vi "Pure Tones.vi"(0 "Amplitude (V)":dbl=1.0 max=19.0 step=1.0, 1 "Frequency (Hz)":dbl=4000.0 min=400.0 max=60000.0 step=10.0, 2 "Stimulation freq (stim/sec)":u32=20, 3 "Fs (#S/s)":dbl=200000.0) -> (4 "Signal duration (ms)":dbl, 5 "Stimulus Waveform":waveform(dbl)(graph), 6 "Stimulus duration (ms)":dbl, 7 "Delay (ms)":dbl=1.0, 8 "Signal duration (#S)":dbl)   [LabVIEW 2014]
uses:
  <vilib>/Analysis/1siggen.llb/Ramp Pattern by Samples.vi
  <vilib>/Analysis/NI_AALBase.lvlib
panel:
  out "Amplitude (1/10 V)":dbl
  out "Phase 1 (degrees)":dbl
  out "Plateu duration (#S)":dbl
  out "Ramp duration (#S)":dbl
  in  "start":dbl
  out "end":dbl
  out "Delay (#S)":dbl
  out "Frecuency (cycles/#S)":dbl
  in  "Plateu duration (ms)":dbl=10.0
  in  "Ramp duration (ms)":dbl=1.0
  # "Stimulus Configuration"
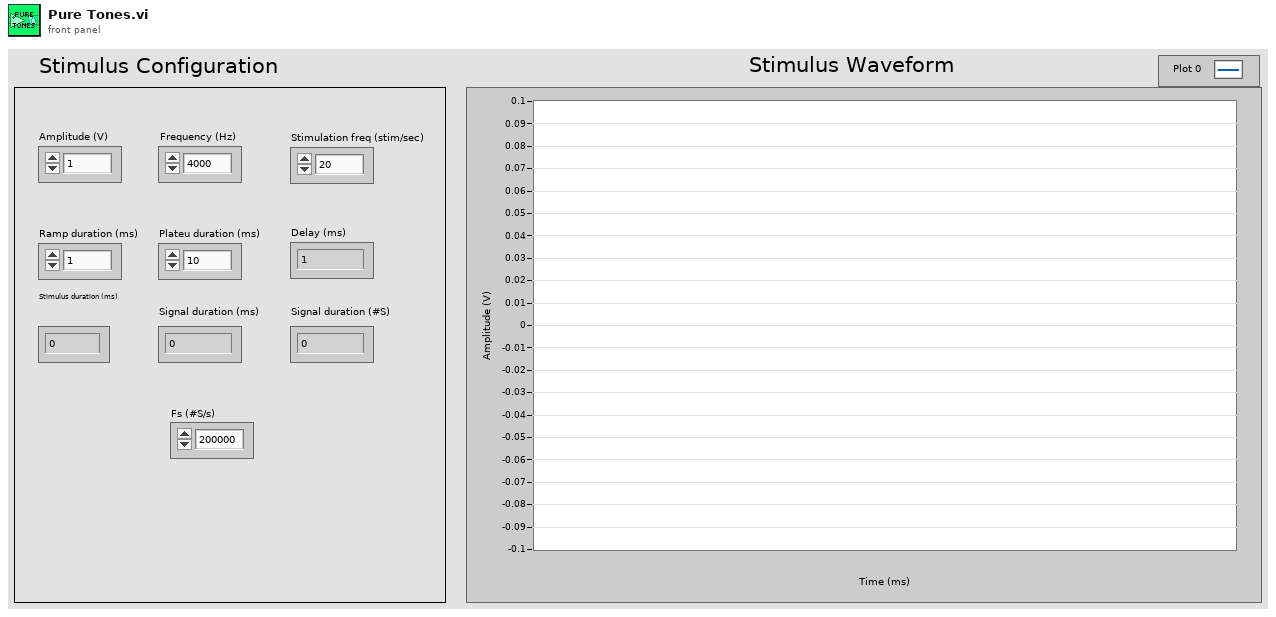
[diagram p1: front panel]
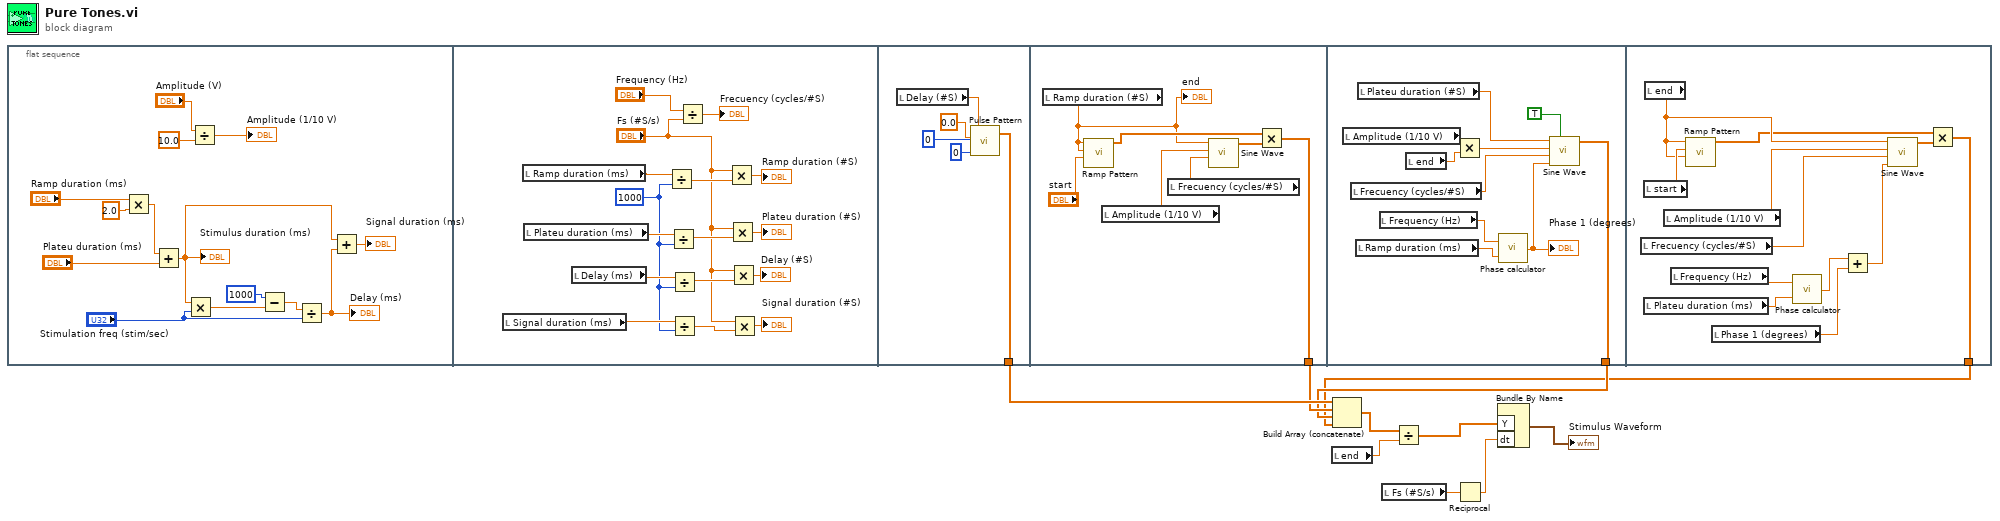
[diagram p0: block diagram]
diagram:
  n1 = flat-sequence {
    tunnel: [w41] -> w9
    tunnel: [w47] -> w8
    tunnel: [w53] -> w7
    tunnel: [w63] -> w6
    frame #0 {
      n2 = Multiply(x="Ramp duration (ms)", y=2.0) -> (x*y=w20:dbl)
      n3 = Add(x=w20, y="Plateu duration (ms)") -> (x+y=w12:dbl)
      "Stimulus duration (ms)" <- w12
      n4 = Multiply(x=w12, y="Stimulation freq (stim/sec)") -> (x*y=w16:dbl)
      n5 = Divide(x="Amplitude (V)", y=10.0) -> (x/y=→"Amplitude (1/10 V)":dbl)
      n6 = Subtract(x=1000, y=w16) -> (x-y=w15:dbl)
      n7 = Divide(x=w15, y="Stimulation freq (stim/sec)") -> (x/y=w11:dbl)
      "Delay (ms)" <- w11
      n8 = Add(x=w12, y=w11) -> (x+y=→"Signal duration (ms)":dbl)
    }
    frame #1 {
      w28 = 1000
      n9 = local read "Signal duration (ms)"() -> (w29:dbl)
      n10 = local read "Ramp duration (ms)"() -> (w38:dbl)
      n11 = local read "Plateu duration (ms)"() -> (w35:dbl)
      n12 = local read "Delay (ms)"() -> (w32:dbl)
      n13 = Divide(x=w38, y=w28) -> (x/y=w36:dbl)
      n14 = Divide(x=w35, y=w28) -> (x/y=w34:dbl)
      n15 = Divide(x=w32, y=w28) -> (x/y=w31:dbl)
      n16 = Divide(x=w29, y=w28) -> (x/y=w27:dbl)
      n17 = Divide(x="Frequency (Hz)", y="Fs (#S/s)") -> (x/y=→"Frecuency (cycles/#S)":dbl)
      n18 = Multiply(x="Fs (#S/s)", y=w36) -> (x*y=→"Ramp duration (#S)":dbl)
      n19 = Multiply(x="Fs (#S/s)", y=w34) -> (x*y=→"Plateu duration (#S)":dbl)
      n20 = Multiply(x="Fs (#S/s)", y=w31) -> (x*y=→"Delay (#S)":dbl)
      n21 = Multiply(x="Fs (#S/s)", y=w27) -> (x*y=→"Signal duration (#S)":dbl)
    }
    frame #2 {
      n22 = local read "Delay (#S)"() -> (w45:dbl)
      n23 = call <vilib>:"Pulse Pattern.vi"("width"=0, "delay"=0, "amplitude"=0.0, "samples"=w45) -> ("Pulse Pattern"=w41:dbl[])  [unwired: 1 out]
    }
    frame #3 {
      n24 = local read "Ramp duration (#S)"() -> (w46:dbl)
      "end" <- w46
      n25 = call-poly <vilib>:"Ramp Pattern.vi"("start"="start", "end"=w46, "samples"=w46) -> ("Ramp Pattern"=w48:dbl[])  [unwired: 7 in, 1 out]
      n26 = local read "Amplitude (1/10 V)"() -> (w50:dbl)
      n27 = local read "Frecuency (cycles/#S)"() -> (w51:dbl)
      n28 = call <vilib>:"Sine Wave.vi"("samples"=w46, "amplitude"=w50, "frequency"=w51) -> ("sine wave"=w49:dbl[])  [unwired: 2 in, 2 out]
      n29 = Multiply(x=w48, y=w49) -> (x*y=w47:dbl[])
    }
    frame #4 {
      n30 = local read "Amplitude (1/10 V)"() -> (w61:dbl)
      n31 = local read "Frecuency (cycles/#S)"() -> (w58:dbl)
      n32 = local read "Ramp duration (ms)"() -> (w56:dbl)
      n33 = local read "Plateu duration (#S)"() -> (w62:dbl)
      n34 = local read "Frequency (Hz)"() -> (w57:dbl)
      n35 = local read "end"() -> (w60:dbl)
      n36 = Multiply(x=w61, y=w60) -> (x*y=w59:dbl)
      n37 = call <userlib>:"Phase calculator.vi"("Frequency (Hz)"=w56, "Ramp duration (ms)"=w57) -> ("Phase (degrees)"=w55:dbl)
      "Phase 1 (degrees)" <- w55
      n38 = call <vilib>:"Sine Wave.vi"("samples"=w62, "amplitude"=w59, "frequency"=w58, "phase in"=w55, "reset phase"=TRUE) -> ("sine wave"=w53:dbl[])  [unwired: 2 out]
    }
    frame #5 {
      n39 = local read "Frecuency (cycles/#S)"() -> (w69:dbl)
      n40 = local read "start"() -> (w74:dbl)
      n41 = local read "Plateu duration (ms)"() -> (w68:dbl)
      n42 = local read "end"() -> (w73:dbl)
      n43 = local read "Amplitude (1/10 V)"() -> (w72:dbl)
      n44 = local read "Frequency (Hz)"() -> (w67:dbl)
      n45 = call-poly <vilib>:"Ramp Pattern.vi"("start"=w73, "end"=w74, "samples"=w73) -> ("Ramp Pattern"=w70:dbl[])  [unwired: 7 in, 1 out]
      n46 = local read "Phase 1 (degrees)"() -> (w66:dbl)
      n47 = call <userlib>:"Phase calculator.vi"("Frequency (Hz)"=w68, "Ramp duration (ms)"=w67) -> ("Phase (degrees)"=w65:dbl)
      n48 = Add(x=w65, y=w66) -> (x+y=w64:dbl)
      n49 = call <vilib>:"Sine Wave.vi"("samples"=w73, "amplitude"=w72, "frequency"=w69, "phase in"=w64) -> ("sine wave"=w71:dbl[])  [unwired: 1 in, 2 out]
      n50 = Multiply(x=w70, y=w71) -> (x*y=w63:dbl[])
    }
  }
  n51 = local read "end"() -> (w4:dbl)
  n52 = Build Array (concatenate)(w9, w8, w7, w6) -> (w5:dbl[])
  n53 = local read "Fs (#S/s)"() -> (w1:dbl)
  n54 = Divide(x=w5, y=w4) -> (x/y=w3:dbl[])
  n55 = Reciprocal(x=w1) -> (1/x=w2:dbl)
  n56 = Bundle By Name("Y"=w3, "dt"=w2) -> (→"Stimulus Waveform":waveform(dbl))  [unwired: 1 in]
